vi "Intro To LV2OO Style Globals.vi"() -> ()   [LabVIEW 2014]
uses:
  Data/Data.lvclass
  Act_Increment All/Act_Increment All.lvclass
  Core Components/Act_Append Many/Act_Append Many.lvclass
  Core Components/Act_Set One/Act_Set One.lvclass
  Core Components/Act_Delete One/Act_Delete One.lvclass
  Core Components/Act_Get One/Act_Get One.lvclass
panel:
  out "Pass?":bool
  # "This VI demos a new way to write LV2 style globals. These \"globals\" are executable VIs with a loop that only runs once on each call and an uninitialized shift register on that loop that remembers the value from call to call. See LV's online documentation for more details. \n\nThe revised version uses LabVIEW classes to dramatically extend the power and performance of the LV2 style global. Because this global is Object Oriented, I've termed it an LV2OO style global.\n\nFurther comments on block diagram and throughout subVIs."
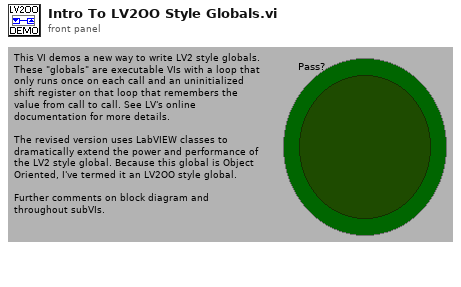
[diagram p1: front panel]
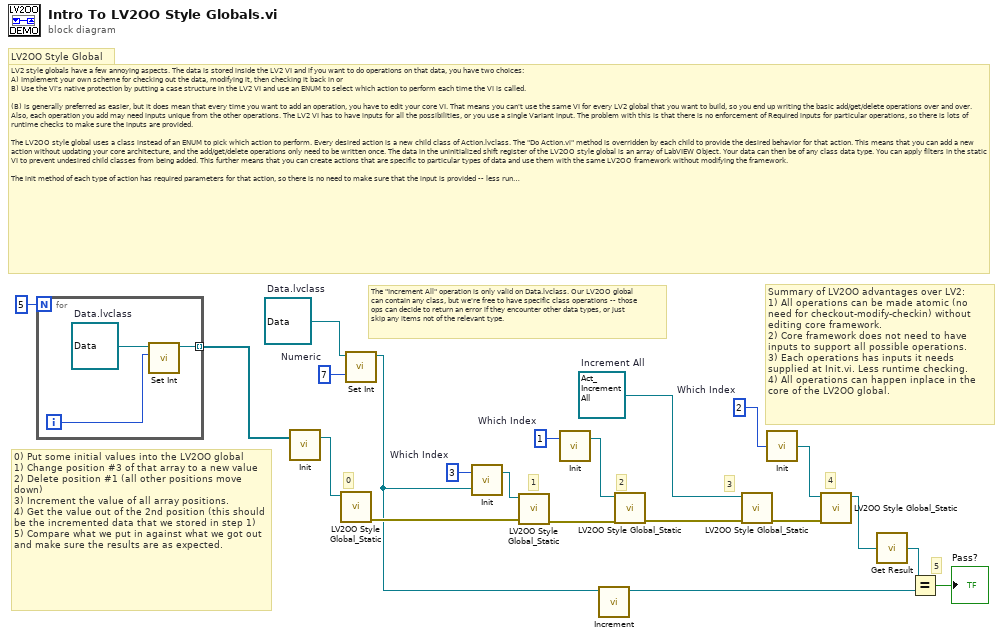
[diagram p0: block diagram]
diagram:
  w1 = refnum<class "Act_Increment All.lvclass"> refnum  # Increment All
  w10 = 2  # Which Index
  w13 = 1  # Which Index
  w16 = 3  # Which Index
  w17 = 7  # Numeric
  w18 = refnum<class "Data.lvclass"> refnum  # Data.lvclass
  # "Summary of LV2OO advantages over LV2:\n1) All operations can be made atomic (no need for checkout-modify-checkin) without editing core framework.\n2) Core framework does not need to have inputs to support all possible operations.\n3) Each operations has inputs it needs supplied at Init.vi. Less runtime checking.\n4) All operations can happen inplace in the core of the LV2OO global."
  # "The \"Increment All\" operation is only valid on Data.lvclass. Our LV2OO global\ncan contain any class, but we're free to have specific class operations -- those\nops can decide to return an error if they encounter other data types, or just \nskip any items not of the relevant type."
  # "5"
  # "4"
  # "2"
  # "1"
  # "0"
  # "3"
  # "0) Put some initial values into the LV2OO global\n1) Change position #3 of that array to a new value\n2) Delete position #1 (all other positions move down)\n3) Increment the value of all array positions.\n4) Get the value out of the 2nd position (this should be the incremented data that we stored in step 1)\n5) Compare what we put in against what we got out and make sure the results are as expected."
  # "LV2 style globals have a few annoying aspects. The data is stored inside the LV2 VI and if you want to do operations on that data, you have two choices: \nA) Implement your own scheme for checking out the data, modifying it, then checking it back in or\nB) Use the VI's native protection by putting a case structure in the LV2 VI and use an ENUM to select which action to perform each time the VI is called.\n\n(B) is generally preferred as easier, but it does mean that every time you want to add an operation, you have to edit your core VI. That means you can't use the same VI for every LV2 global that you want to build, so you end up writing the basic add/get/delete operations over and over. Also, each operation you add may need inputs unique from the other operations. The LV2 VI has to have inputs for all the possibilities, or you use a single Variant input. The problem with this is that there is no enforcement of Required inputs for particular operations, so there is lots of runtime checks to make sure the inputs are provided.  \n\nThe LV2OO style global uses a class instead of an ENUM to pick which action to perform. Every desired action is a new child class of Action.lvclass. The \"Do Action.vi\" method is overridden by each child to provide the desired behavior for that action. This means that you can add a new action without updating your core architecture, and the add/get/delete operations only need to be written once. The data in the uninitialized shift register of the LV2OO style global is an array of LabVIEW Object. Your data can then be of any class data type. You can apply filters in the static VI to prevent undesired child classes from being added. This further means that you can create actions that are specific to particular types of data and use them with the same LV2OO framework without modifying the framework.\n\nThe init method of each type of action has required parameters for that action, so there is no need to make sure that the input is provided -- less runtime error checking!"
  # "LV2OO Style Global"
  n1 = for {
    N: 5 -> [_]
    tunnel: [w22] -> w20 mode=indexing
    i -> [w23]
    w24 = refnum<class "Data.lvclass"> refnum  # Data.lvclass
    n2 = call-dynamic "Set Int.vi"("Numeric"=w23, "Data in"=w24) -> ("Data out"=w22:refnum<class "Data.lvclass">)  [unwired: 8 in, 1 out]
  }
  n3 = call "Init.vi"("Append These"=w20) -> ("Action out"=w19:refnum<class "Act_Append Many.lvclass">)  [unwired: 2 in]
  n4 = call "LV2OO Style Global_Static.vi"("Action in"=w19) -> ("error out"=w15:errorcluster)  [unwired: 5 in, 1 out]
  n5 = call-dynamic "Set Int.vi"("Numeric"=w17, "Data in"=w18) -> ("Data out"=w5:refnum<class "Data.lvclass">)  [unwired: 8 in, 1 out]
  n6 = call "Init.vi"("Value"=w5, "Which Index"=w16) -> ("Action out"=w14:refnum<class "Act_Set One.lvclass">)  [unwired: 1 in]
  n7 = call "LV2OO Style Global_Static.vi"("error in (no error)"=w15, "Action in"=w14) -> ("error out"=w12:errorcluster)  [unwired: 4 in, 1 out]
  n8 = call "Init.vi"("Which Index"=w13) -> ("Act_Delete One.lvclass"=w11:refnum<class "Act_Delete One.lvclass">)  [unwired: 2 in]
  n9 = call-dynamic "Increment.vi"("Data in"=w5) -> ("Data out"=w4:refnum<class "Data.lvclass">)  [unwired: 9 in, 1 out]
  n10 = call "LV2OO Style Global_Static.vi"("error in (no error)"=w12, "Action in"=w11) -> ("error out"=w2:errorcluster)  [unwired: 4 in, 1 out]
  n11 = call "LV2OO Style Global_Static.vi"("error in (no error)"=w2, "Action in"=w1) -> ("error out"=w3:errorcluster)  [unwired: 4 in, 1 out]
  n12 = call "Init.vi"("Which Index"=w10) -> ("Action out"=w9:refnum<class "Act_Get One.lvclass">)
  n13 = call "LV2OO Style Global_Static.vi"("error in (no error)"=w3, "Action in"=w9) -> ("Action out"=w8:refnum<class "Act_Get One.lvclass">)  [unwired: 4 in, 1 out]
  n14 = call "Get Result.vi"("Act_Get One.lvclass"=w8) -> ("Result"=w7:refnum<class>)
  n15 = Equal?(x=w7, y=w4) -> (x = y?=→"Pass?":bool)
